vi "Measure.vi"(8 "error in (no error)":errorcluster, 9 "measurement configuration":variant, 10 "measure call context in":refnum<class "Measure Call Context.lvclass">, 11 "measurement plugin in":refnum<class "FPT_Compression.lvclass">) -> (0 "error out":errorcluster, 1 "measurement results":variant, 2 "measure call context out":refnum<class "Measure Call Context.lvclass">, 3 "measurement plugin out":refnum<class "FPT_Compression.lvclass">)   [LabVIEW 2023, in "FPT_Compression.lvclass"]
uses:
  FPT_Compression.lvclass
  <vilib>/Plug-In SDKs/Measurements/Measure Call Context/Measure Call Context.lvclass
  Measurement Configuration.ctl
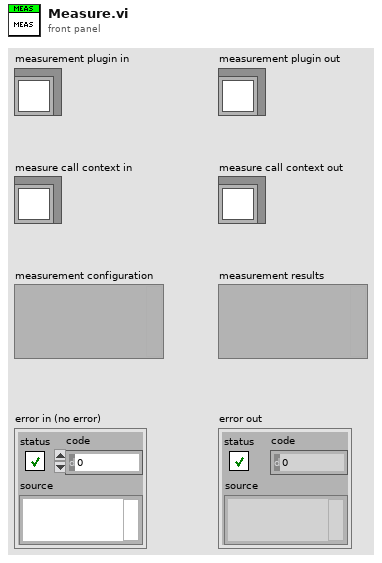
[diagram p1: front panel]
types:
  T1 = typedef "FPT_Compression.lvclass/Measurement Configuration.ctl" = cluster{"Automation Test":bool, "Power sequencing file path":string, "SMU name":string, "SMU channel":string, "RFSG name":string, "RFSG port":string, "RFSG attenuation mode":enum32{"<None>", "Constant Attenuation", "s2p File"}, "RFSG external attenuation (dB)":dbl, "RFSG s-parameters orientation":enum32{"Port1 Towards DUT", "Port2 Towards DUT"}, "RFSG s2p file path":string, "RFmx name":string, "RFmx port":string, "RFmx attenuation mode":enum32{"<None>", "Constant Attenuation", "s2p File"}, "RFmx external attenuation (dB)":dbl, "RFmx attenuation path name":string, "RFmx s-parameters orientation":enum32{"Port1 Towards DUT", "Port2 Towards DUT"}, "RFmx attenuation s2p path name":string, "RFmx s2p file path":string, "Compression_Expected DUT Gain (dB)":dbl, "Compression_Max Linear Range (dBm)":dbl, "Compression_Compression Point (dB)":dbl, "Compression_Target Pin (dBm)":dbl, "Compression_RFSG Frequency Start (Hz)":dbl, "Compression_RFSG Frequency Stop (Hz)":dbl, "Compression_RFSG Number of Frequency Step":i32, "Compression_RFSG Power Start (dBm)":dbl, "Compression_RFSG Power Stop(dBm)":dbl, "Compression_RFSG Power Step Size (dB)":dbl, "Compression_RBW (Hz)":dbl, "Compression_RF Measurement Interval (s)":dbl, "Compression_DC Measurement Interval (s)":dbl, "Compression_Stimulus Mode":enum32{"Constant Power and RF", "Constant Power and Pulsed RF", "Pulsed Power and RF"}, "CP_CW_DC Source Delay (s)":dbl, "CP_PRF_DC Source Delay (s)":dbl, "CP_PRF_RFmx Trigger Delay (s)":dbl, "CP_PRF_RF Pulse Width (s)":dbl, "CP_PRF_PRI (s)":dbl, "PP_PRF_DC Source Delay (s)":dbl, "PP_PRF_RFmx Trigger Delay (s)":dbl, "PP_PRF_RF Pulse Width (s)":dbl, "PP_PRF_PRI (s)":dbl, "PP_PRF_DC Pulse Width (s)":dbl, "PP_PRF_ON Current Limit (A)":dbl, "PP_PRF_Bias Voltage Level (V)":dbl, "PP_PRF_Bias Current Limit (A)":dbl}
  T2 = typedef "FPT_Compression.lvclass/Measurement Results.ctl" = cluster{"Status":string, "per Freq Plot Names":string[], "Linear Gain vs Freq":dbl[][], "OPxdB vs Freq":dbl[][], "Pout@Pin vs Freq":dbl[][], "Gain@Pin vs Freq":dbl[][], "PAE@Pin vs Freq":dbl[][], "Pout vs Pin per Freq":dbl[][], "Gain vs Pin per Freq":dbl[][], "PAE vs Pin per Freq":dbl[][], "Pout@Pin (Mean)":dbl, "Gain@Pin (Mean)":dbl, "PAE@Pin (Mean)":dbl, "Linear Gain (Mean)":dbl, "OPxdB (Mean)":dbl}
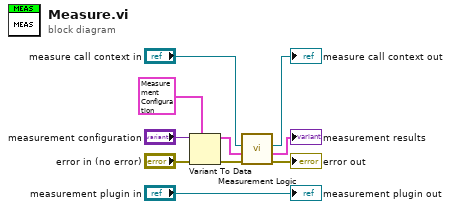
[diagram p0: block diagram]
diagram:
  n1 = Variant To Data(error in="error in (no error)", type=T1 {"Automation Test"=FALSE, "Power sequencing file path"="Lorem ipsum dolor sit", "SMU name"="", "SMU channel"="0", "RFSG name"="5842_0", "RFSG port"="", "RFSG attenuation mode"=enum."s2p File", "RFSG external attenuation (dB)"=64.0, "RFSG s-parameters orientation"=enum."Port1 Towards DUT", "RFSG s2p file path"="", "RFmx name"="Lorem ipsum dolor sit", "RFmx port"="", "RFmx attenuation mode"=enum."Constant Attenuation", "RFmx external attenuation (dB)"=-64.0, "RFmx attenuation path name"="", "RFmx s-parameters orientation"=enum."Port2 Towards DUT", "RFmx attenuation s2p path name"="", "RFmx s2p file path"="", "Compression_Expected DUT Gain (dB)"=17.5, "Compression_Max Linear Range (dBm)"=-10.0, "Compression_Compression Point (dB)"=1.0, "Compression_Target Pin (dBm)"=1.0, "Compression_RFSG Frequency Start (Hz)"=10000000000.0, "Compression_RFSG Frequency Stop (Hz)"=18000000000.0, "Compression_RFSG Number of Frequency Step"=10, "Compression_RFSG Power Start (dBm)"=-20.0, "Compression_RFSG Power Stop(dBm)"=1.0, "Compression_RFSG Power Step Size (dB)"=4.0, "Compression_RBW (Hz)"=5000000.0, "Compression_RF Measurement Interval (s)"=0.001, "Compression_DC Measurement Interval (s)"=0.001, "Compression_Stimulus Mode"=enum."Constant Power and RF", "CP_CW_DC Source Delay (s)"=0.0, "CP_PRF_DC Source Delay (s)"=0.0, "CP_PRF_RFmx Trigger Delay (s)"=0.0, "CP_PRF_RF Pulse Width (s)"=0.0001, "CP_PRF_PRI (s)"=0.001, "PP_PRF_DC Source Delay (s)"=0.0, "PP_PRF_RFmx Trigger Delay (s)"=0.0, "PP_PRF_RF Pulse Width (s)"=0.0001, "PP_PRF_PRI (s)"=0.001, "PP_PRF_DC Pulse Width (s)"=0.0008, "PP_PRF_ON Current Limit (A)"=2.0, "PP_PRF_Bias Voltage Level (V)"=0.0, "PP_PRF_Bias Current Limit (A)"=0.2} ("measurement configuration"), Variant="measurement configuration") -> (data=w1:T1, error out=w7:errorcluster)
  n2 = call "Measurement Logic.vi"("error in"=w7, "measurement configuration"=w1, "measure call context in"="measure call context in") -> ("error out"=→"error out":errorcluster, "measurement results"=→"measurement results":T2, "measure call context out"=→"measure call context out":refnum<class "Measure Call Context.lvclass">)  [unwired: 6 in]
  "measurement plugin out" <- "measurement plugin in"
